vi "appendSummary.vi"(8 "error in (no error)":errorcluster, 11 "TestDataLog in":refnum<class "TestDataLog.lvclass">) -> (0 "error out":errorcluster, 3 "TestDataLog out":refnum<class "TestDataLog.lvclass">)   [LabVIEW 2015, in "TestDataLog.lvclass"]
uses:
  TestDataLog.lvclass
  <userlib>/Common/Log/Log/Log.lvclass/Log.ctl
  TestDataLog.lvclass/TestDataLog.ctl
  <userlib>/Common/Log/Log/Log.lvclass
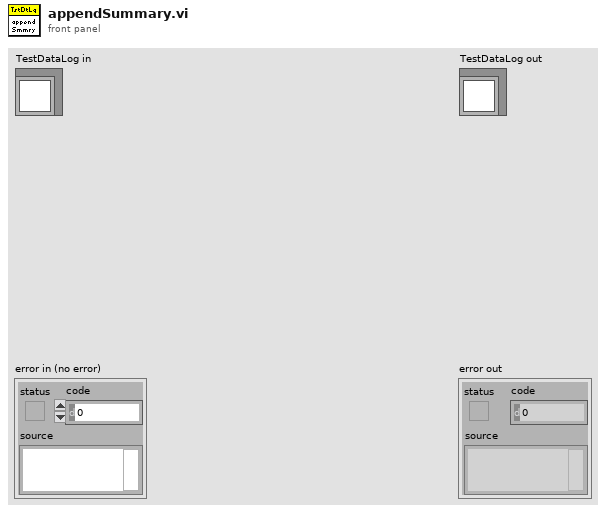
[diagram p1: front panel]
types:
  T1 = typedef "Log.lvlib/Log.ctl" = cluster{"Log Directory":path, "Log Filename Base":string, "Max records per file":u32, "Comment":string}
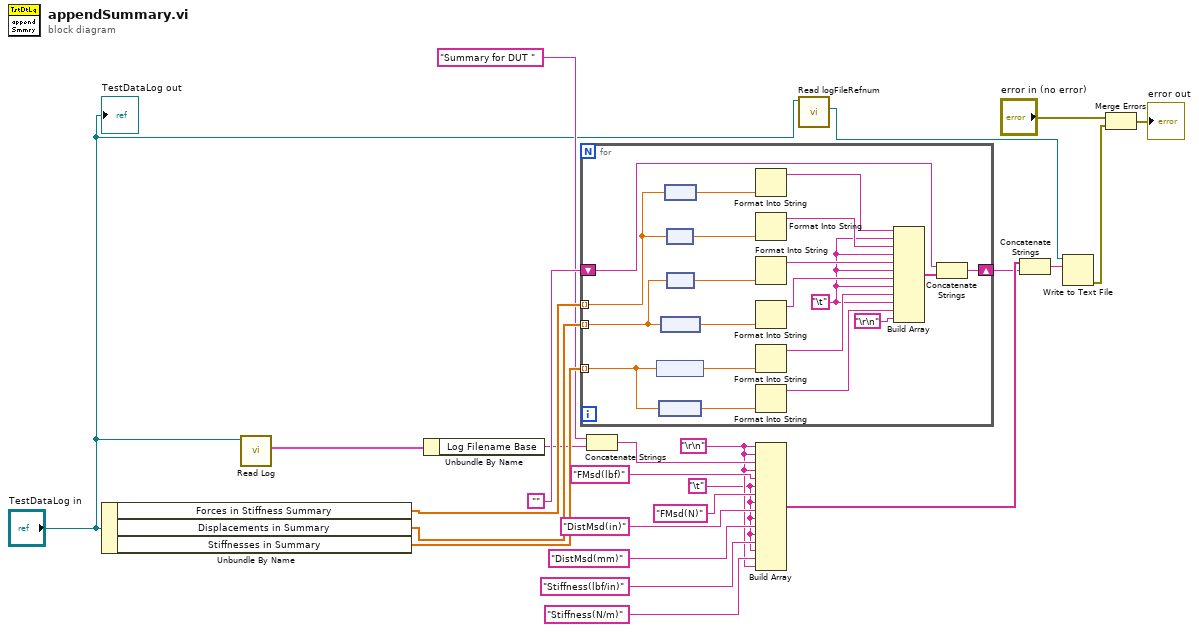
[diagram p0: block diagram]
diagram:
  w1 = "\t"
  w2 = "\r\n"
  n1 = Unbundle By Name("TestDataLog in") -> ("Forces in Stiffness Summary"=w18:dbl[unit][], "Displacements in Summary"=w17:dbl[unit][], "Stiffnesses in Summary"=w16:dbl[unit][])
  n2 = call <userlib>:"Read Log.vi"("Log in"="TestDataLog in") -> ("Log"=w8:T1)  [unwired: 9 in, 1 out]
  n3 = Unbundle By Name(w8) -> ("Log Filename Base"=w7:string)
  n4 = for {
    tunnel: w18 -> [w38] mode=indexing
    tunnel: w17 -> [w37] mode=indexing
    tunnel: w16 -> [w36] mode=indexing
    shift-right: [w25] -> w13
    shift-left: "" -> [w27]
    w29 = "\t"
    n5 = node(w36) -> (w39:dbl)
    n6 = node(w36) -> (w40:dbl)
    n7 = node(w37) -> (w42:dbl)
    n8 = node(w38) -> (w43:dbl)
    n9 = node(w38) -> (w44:dbl)
    n10 = node(w37) -> (w41:dbl)
    n11 = Format Into String(w43) -> (resulting string=w35:string)  [unwired: 3 in, 1 out]
    n12 = Format Into String(w44) -> (resulting string=w34:string)  [unwired: 3 in, 1 out]
    n13 = Format Into String(w41) -> (resulting string=w33:string)  [unwired: 3 in, 1 out]
    n14 = Format Into String(w42) -> (resulting string=w32:string)  [unwired: 3 in, 1 out]
    n15 = Format Into String(w39) -> (resulting string=w31:string)  [unwired: 3 in, 1 out]
    n16 = Format Into String(w40) -> (resulting string=w30:string)  [unwired: 3 in, 1 out]
    n17 = Build Array(w35, w29, w34, w29, w33, w29, w32, w29, w31, w29, w30, "\r\n") -> (w26:string[])
    n18 = Concatenate Strings(w27, w26) -> (w25:string)
  }
  n19 = Concatenate Strings("Summary for DUT ", w7) -> (w5:string)
  n20 = Build Array(w2, w2, w5, w2, "FMsd(lbf)", w1, "FMsd(N)", w1, "DistMsd(in)", w1, "DistMsd(mm)", w1, "Stiffness(lbf/in)", w1, "Stiffness(N/m)", w2) -> (w15:string[])
  n21 = call <userlib>:"Read logFileRefnum.vi"("Log in"="TestDataLog in") -> ("logFileRefnum"=w3:refnum<file>)  [unwired: 9 in, 1 out]
  n22 = Concatenate Strings(w15, w13) -> (w9:string)
  n23 = Write to Text File(file (use dialog)=w3, text=w9) -> (error out=w11:errorcluster)  [unwired: 2 in, 2 out]
  n24 = Merge Errors("error in (no error)", w11) -> (→"error out":errorcluster)
  "TestDataLog out" <- "TestDataLog in"
